vi "Pre Launch Init.vi"(11 "Actor_AFG in":refnum<class "Actor_AFG.lvclass">) -> (0 "error out":errorcluster, 3 "Actor_AFG out":refnum<class "Actor_AFG.lvclass">)   [LabVIEW 2020, in "Actor_AFG.lvlib" / "Actor_AFG.lvclass"]
doc: "(<B>Filename</B>: Actor Framework.lvlib:Actor.lvclass:Pre Launch Init.vi)\n\nDefines behavior that occurs after the Launch Nested Actor method is invoked but before the actor's Actor Core method begins running.\n\nBy default, this method does nothing. A descendant class may override it to define behavior."
uses:
  Actor_AFG.lvclass
  C:/Program Files/National Instruments/LabVIEW 2020/vi.lib/ActorFramework/Actor/Actor.lvclass
  <vilib>/ActorFramework/Actor/Actor.lvclass/Actor.ctl
  Actor_AFG.lvclass/Actor_AFG.ctl
  AFG_Event.ctl
  <vilib>/ActorFramework/Actor/Actor.lvclass
  <instrlib>/Tektronix AFG 3000 Series/Tektronix AFG 3000 Series.lvlib
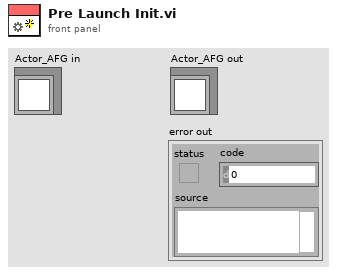
[diagram p1: front panel]
types:
  T1 = typedef "Actor_AFG.lvlib/Actor_AFG.lvclass/AFG_Event.ctl" = enum16{"General Event", "Inited", "Output", "Waveform Set", "Error"}
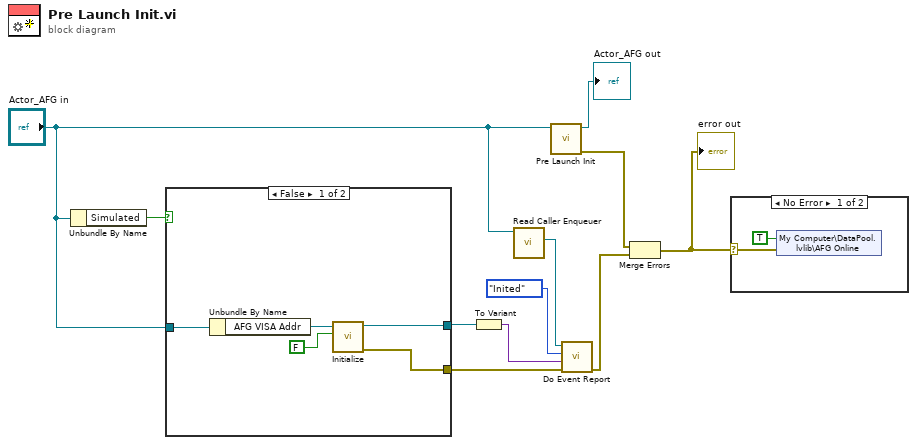
[diagram p0: block diagram]
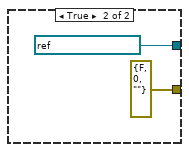
[diagram p3: hidden frame]
diagram:
  n1 = Unbundle By Name("Actor_AFG in") -> ("Simulated"=w10:bool)
  n2 = case shown="False" w10 {
    tunnel: "Actor_AFG in" -> [w16 _]
    tunnel: [w14 refnum<visa-resource-name> "Simulated AFG" ("VISA resource name out")] -> w5
    tunnel: [w13 errorcluster {"status"=FALSE, "code"=0, "source"=""} ("error out")] -> w8
    frame False {
      n3 = Unbundle By Name(w16) -> ("AFG VISA Addr"=w15:refnum<visa-resource-name>)
      n4 = call <instrlib>:"Initialize.vi"("ID Query (True)"=FALSE, "VISA resource name"=w15) -> ("error out"=w13:errorcluster, "VISA resource name out"=w14:refnum<visa-resource-name>)  [unwired: 8 in]
    }
    frame True {
    }
  }
  n5 = To Variant(anything=w5) -> (Variant=w4:variant)
  n6 = call <vilib>:"Read Caller Enqueuer.vi"("Actor"="Actor_AFG in") -> ("Caller Enqueuer"=w6:refnum<class "Message Enqueuer.lvclass">)  [unwired: 10 in]
  n7 = call-parent "Pre Launch Init.vi"("Actor in"="Actor_AFG in") -> ("error out"=w2:errorcluster, "Actor out"=→"Actor_AFG out":refnum<class "Actor_AFG.lvclass">)  [unwired: 9 in]
  n8 = call "Do Event Report.vi"("error in (no error)"=w8, "Event Data"=w4, "Report Events"=AFG_Event."Inited", "Caller Enqueuer"=w6) -> ("error out"=w3:errorcluster)  [unwired: 6 in, 1 out]
  n9 = Merge Errors(w2, w3) -> (w1:errorcluster)
  "error out" <- w1
  n10 = case shown="No Error" w1 {
    selector: w1 -> [w20 _]
    frame No Error {
      n11 = shared-variable "My Computer\\DataPool.lvlib\\AFG Online"(TRUE ("AFG Online"), error in=w20) -> ()  [unwired: 1 out]
    }
    frame Error {
    }
  }
